vi "Untitled 1.vi"() -> ()   [LabVIEW 2016]
uses:
  Control 2.ctl
  Control 1.ctl
  <vilib>/Instr/_visa.llb/VISA Configure Serial Port (Instr).vi
panel:
  in  "Задать текущее положение нулевым":T1
  out "положение шд":T2 scale=-10.0..190.0
  out "минуты":string
  out "градусы, минуты":string
  in  "Установка минут":i32 min=0 max=11400
  out "положение в мин 1":i32
  in  "Stop двигатель":bool
  in  "Вернуться в нулевое положение":bool
  in  "Вращение по минутам -":bool
  in  "Вращение по минутам +":bool
  in  "stop":bool
  out "4":i32
  out "3":i32
  out "2":i32
  out "1":i32
  in  "Выберете порт":refnum<visa-resource-name>="COM1"
  # "Текущее\nположение:"
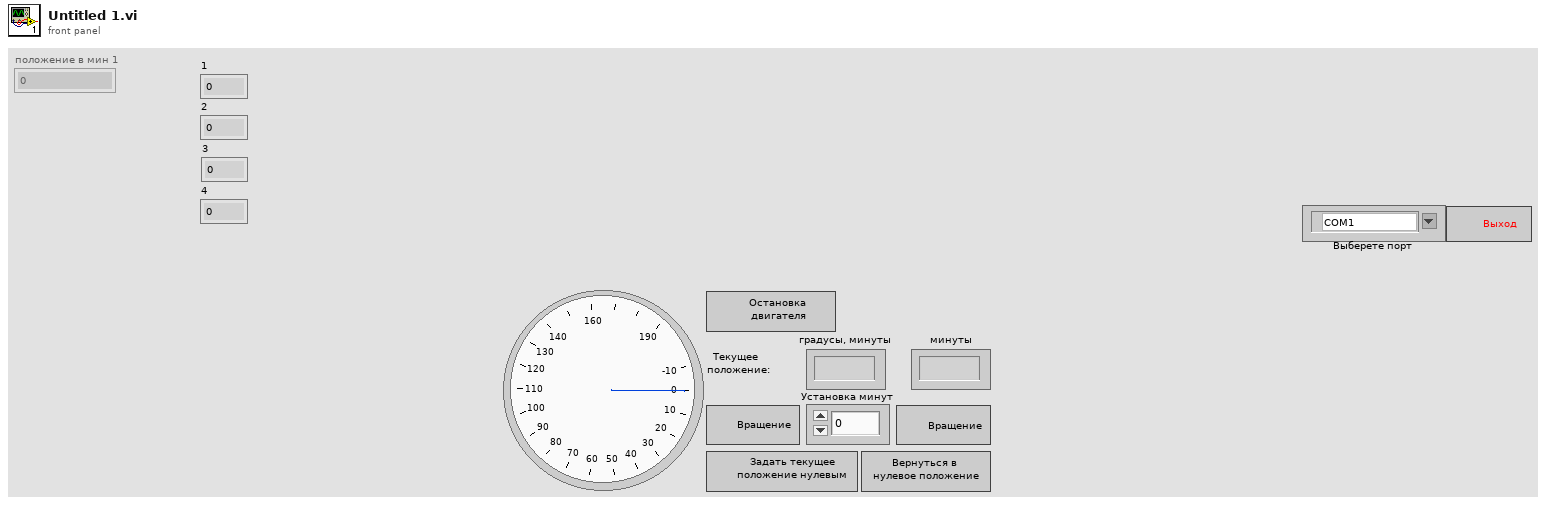
[diagram p1: front panel]
types:
  T1 = typedef "Control 1.ctl" = bool
  T2 = typedef "Control 2.ctl" = i32
  T3 = enum16{"open", "replace", "create", "open or create", "replace or create", "replace or create with confirmation"}
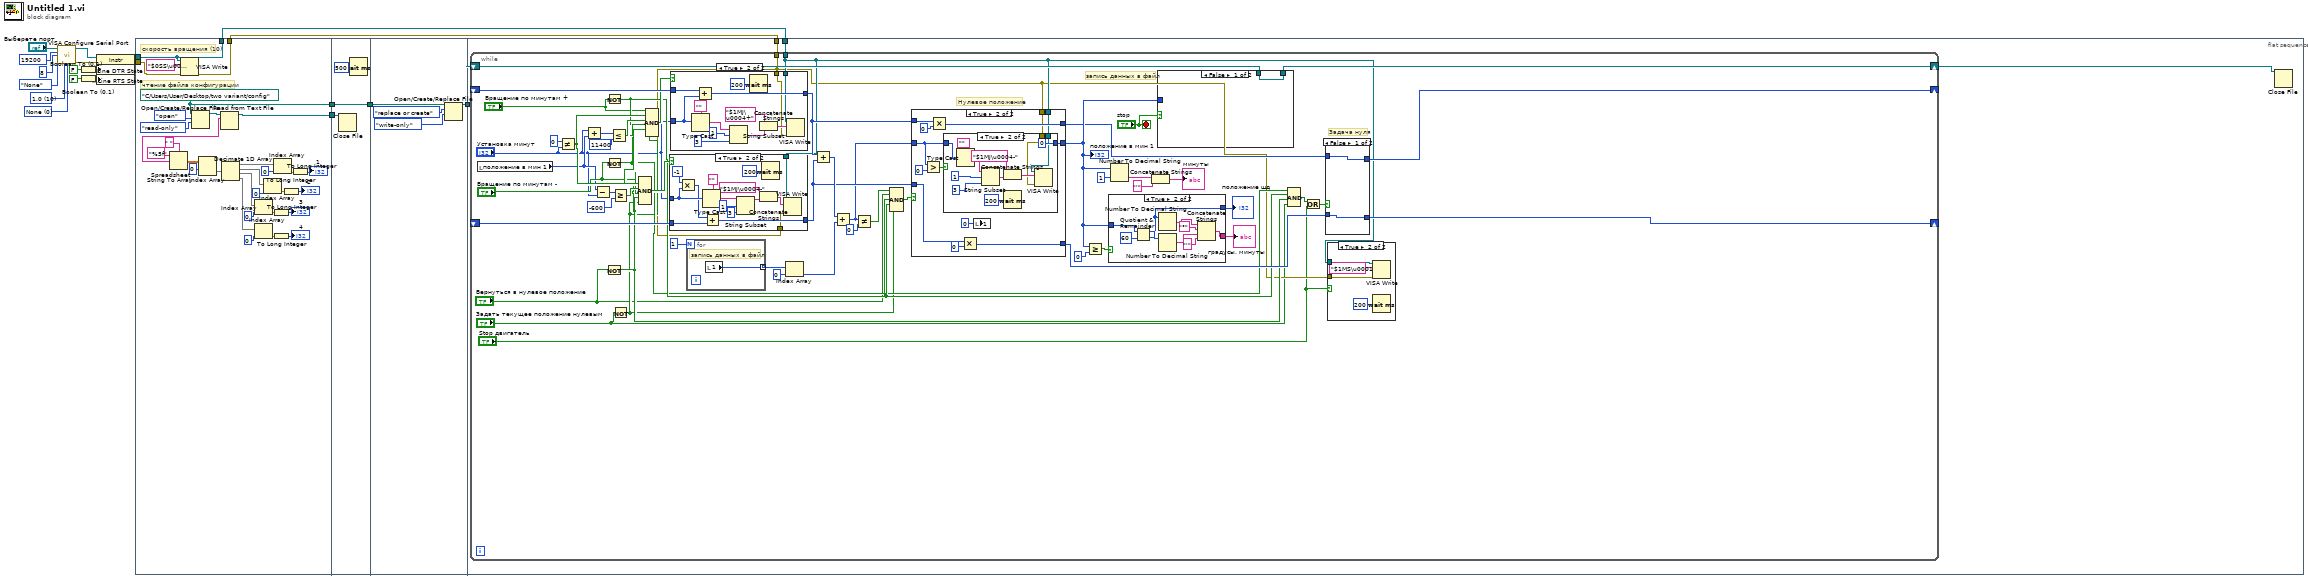
[diagram p0: block diagram]
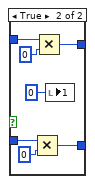
[diagram p3: hidden frame]
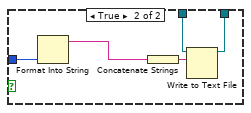
[diagram p4: hidden frame]
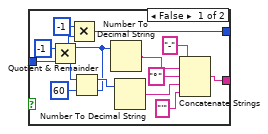
[diagram p5: hidden frame]
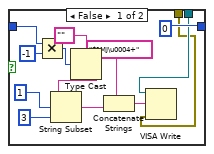
[diagram p7: hidden frame]
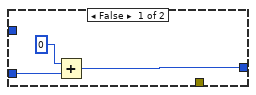
[diagram p8: hidden frame]
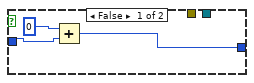
[diagram p9: hidden frame]
diagram:
  w9 = u16 0 items=["None"=0, "XON/XOFF"=1, "RTS/CTS"=2, "DTR/DSR"=4] ("Контроль переполнения")
  w10 = u16 10 items=["1.0"=10, "1.5"=15, "2.0"=20] ("Стоповый бит")
  w13 = u32 19200 items=["9600"=9600, "19200"=19200, "38400"=38400, "57600"=57600] ("Скорость обмена данными")
  n1 = call-poly "VISA Configure Serial Port"("VISA resource name"="Выберете порт", "baud rate (9600)"=w13, "data bits (8)"=u16 8 ("Число бит на символ"), "parity (0:none)"=enum16{"None", "Odd", "Even", "Mark", "Space"}."None" ("Контроль чётности"), "stop bits (10: 1 bit)"=w10, "flow control (0:none)"=w9) -> ("VISA resource name out"=w18:refnum<visa-resource-name>, "error out"=w17:errorcluster)  [unwired: 8 in]
  n2 = Boolean To (0,1)(Boolean=FALSE ("DTR Write")) -> (0, 1=w19:i16)
  n3 = Boolean To (0,1)(Boolean=FALSE ("DTR Write")) -> (0, 1=w20:i16)
  n4 = property class="Instr"(reference=w18, error in=w17, "Serial Settings:Modem Line Settings:Line DTR State"=w19, "Serial Settings:Modem Line Settings:Line RTS State"=w20) -> (reference out=w8:refnum<visa-resource-name>, error out=w7:errorcluster)
  n5 = flat-sequence {
    tunnel: w8 -> [w23]
    tunnel: w7 -> [w22]
    tunnel: [w24] -> w6
    tunnel: [w23] -> w1
    tunnel: [w22] -> w2
    tunnel: [w21] -> w5
    tunnel: w6 -> [w52]
    tunnel: w5 -> [w51]
    tunnel: [w51] -> w4
    tunnel: w4 -> [w55]
    tunnel: [w54] -> w3
    tunnel: w3 -> [w61]
    tunnel: w2 -> [w58]
    tunnel: w1 -> [w59]
    frame #0 {
      w21 = path "C:/Users/User/Desktop/two variant/config"
      # "чтение файла конфигурации"
      # "скорость вращения (10)"
      n6 = VISA Write(VISA resource name=w23, write buffer="$0SS\u0001\u0010", error in (no error)=w22) -> ()  [unwired: 3 out]
      n7 = Open/Create/Replace File(file path (use dialog)=w21, operation (0:open)=T3."open", access (0:read/write)=enum16{"read/write", "read-only", "write-only"}."read-only") -> (refnum out=w47:refnum<file>)  [unwired: 3 in, 2 out]
      n8 = Read from Text File(file (use dialog)=w47) -> (refnum out=w24:refnum<file>, text=w34:string)  [unwired: 3 in, 2 out]
      n9 = Spreadsheet String To Array(delimiter (Tab)=" ", format string="%5f", spreadsheet string=w34) -> (array=w44:dbl[][])  [unwired: 1 in]
      n10 = Index Array(array=w44, index (row)=0 ("index")) -> (element=w42:dbl[])  [unwired: 1 in]
      n11 = Decimate 1D Array(w42) -> (w39:dbl[], w30:dbl[], w29:dbl[], w25:dbl[])
      n12 = Index Array(array=w29, index=0) -> (element=w32:dbl)
      n13 = Index Array(array=w25, index=0) -> (element=w27:dbl)
      n14 = Index Array(array=w30, index=0) -> (element=w38:dbl)
      n15 = To Long Integer(number=w32) -> (32bit integer=→"3":i32)
      n16 = To Long Integer(number=w27) -> (32bit integer=→"4":i32)
      n17 = Index Array(array=w39, index=0) -> (element=w37:dbl)
      n18 = To Long Integer(number=w38) -> (32bit integer=→"2":i32)
      n19 = To Long Integer(number=w37) -> (32bit integer=→"1":i32)
    }
    frame #1 {
      n20 = Close File(refnum=w52) -> ()  [unwired: 1 in, 2 out]
      n21 = Wait (ms)(milliseconds to wait=u32 500) -> ()  [unwired: 1 out]
    }
    frame #2 {
      n22 = Open/Create/Replace File(file path (use dialog)=w55, operation (0:open)=T3."replace or create", access (0:read/write)=enum16{"read/write", "read-only", "write-only"}."write-only") -> (refnum out=w54:refnum<file>)  [unwired: 3 in, 2 out]
    }
    frame #3 {
      n23 = while {
        shift-right: [w85] -> w60
        shift-left: w61 -> [w86]
        shift-right: [w81] -> _
        shift-left: _ -> [w115]
        shift-right: [w80] -> _
        shift-left: _ -> [w109]
        tunnel: w59 -> [w73]
        tunnel: w58 -> [w72]
        stop <- "stop" stop-if-true
        # "Задача нуля"
        # "запись данных в файл"
        # "Нулевое положение"
        n24 = local read "положение в мин 1"() -> (w64:i32)
        n25 = Not Equal?(x=0 ("y"), y="Установка минут") -> (x != y?=w108:bool)
        n26 = Add(x="Установка минут", y=w64) -> (x+y=w113:i32)
        n27 = Subtract(x=w64, y="Установка минут") -> (x-y=w65:i32)
        n28 = Not(x="Вернуться в нулевое положение") -> (.not. x?=w79:bool)
        n29 = Not(x="Вращение по минутам +") -> (.not. x?=w78:bool)
        n30 = Not(x="Вращение по минутам -") -> (.not. x?=w77:bool)
        n31 = Less Or Equal?(x=w113, y=11400) -> (x <= y?=w112:bool)
        n32 = Greater Or Equal?(x=w65, y=-600) -> (x >= y?=w106:bool)
        n33 = Not(x="Задать текущее положение нулевым") -> (.not. x?=w76:T1)
        n34 = Compound Arithmetic op=AND("Вращение по минутам -", w108, w106, w78, w79, w76) -> (w105:T1)
        n35 = Compound Arithmetic op=AND("Вращение по минутам +", w108, w112, w77, w79, w76) -> (w110:T1)
        n36 = case shown="True" w105 {
          tunnel: [w201 w210] -> w95
          tunnel: "Установка минут" -> [_ w205]
          tunnel: w109 -> [w200 w206]
          tunnel: w73 -> [_ w208]
          tunnel: w72 -> [_ w207]
          frame False {
            n37 = Add(x=0, y=w200) -> (x+y=w201:i32)
          }
          frame True {
            n38 = Multiply(x=-1, y=w205) -> (x*y=w204:i32)
            n39 = Type Cast(type="", x=w205) -> (*(type *) &x=w213:string)
            n40 = Add(x=w204, y=w206) -> (x+y=w210:i32)
            n41 = String Subset(string=w213, offset (0)=1, length (rest)=3 ("length (rest)")) -> (substring=w212:string)
            n42 = Concatenate Strings("$1MJ\u0004-" ("write buffer"), w212) -> (w216:string)
            n43 = Wait (ms)(milliseconds to wait=u32 200) -> ()  [unwired: 1 out]
            n44 = VISA Write(VISA resource name=w208, write buffer=w216, error in (no error)=w207) -> ()  [unwired: 3 out]
          }
        }
        n45 = case shown="True" w110 {
          tunnel: [w219 w226] -> w96
          tunnel: "Установка минут" -> [_ w225]
          tunnel: w115 -> [w218 w222]
          tunnel: w73 -> [_ w224]
          tunnel: w72 -> [_ w223]
          frame False {
            n46 = Add(x=0, y=w218) -> (x+y=w219:i32)
          }
          frame True {
            n47 = Type Cast(type="", x=w225) -> (*(type *) &x=w229:string)
            n48 = Add(x=w222, y=w225) -> (x+y=w226:i32)
            n49 = String Subset(string=w229, offset (0)=1, length (rest)=3 ("length (rest)")) -> (substring=w228:string)
            n50 = Wait (ms)(milliseconds to wait=u32 200) -> ()  [unwired: 1 out]
            n51 = Concatenate Strings("$1MJ\u0004+" ("write buffer"), w228) -> (w232:string)
            n52 = VISA Write(VISA resource name=w224, write buffer=w232, error in (no error)=w223) -> ()  [unwired: 3 out]
          }
        }
        n53 = for {
          N: 1 -> [_]
          tunnel: [w199] -> w103 mode=indexing
          # "запись данных в файл"
          n54 = local read "1"() -> (w199:i32)
        }
        n55 = Index Array(array=w103, index=0) -> (element=w101:i32)
        n56 = Add(x=w96, y=w95) -> (x+y=w100:i32)
        n57 = Add(x=w100, y=w101) -> (x+y=w94:i32)
        n58 = Not Equal?(x=w94, y=0) -> (x != y?=w98:bool)
        n59 = Compound Arithmetic op=AND(w98, "Вернуться в нулевое положение", w77, w78, w76) -> (w97:T1)
        n60 = case shown="True" w97 {
          tunnel: [w158 w173] -> w84
          tunnel: [w160 w171] -> w83
          tunnel: [w159 w167] -> w82
          tunnel: w96 -> [w160 w165]
          tunnel: w95 -> [w159 w164]
          tunnel: w94 -> [w158 w163]
          tunnel: w73 -> [_ w162]
          tunnel: w72 -> [_ w161]
          frame False {
          }
          frame True {
            n61 = Greater?(x=w163, y=0) -> (0:w168:bool)
            n62 = Multiply(x=w165, y=0) -> (x*y=w171:i32)
            n63 = case shown="True" w168 {
              tunnel: [0 0] -> w173
              tunnel: w163 -> [w176 w190]
              tunnel: w162 -> [w175 w188]
              tunnel: w161 -> [w174 w189]
              frame False {
                n64 = Multiply(x=w176, y=-1) -> (x*y=w177:i32)
                n65 = Type Cast(type="", x=w177) -> (*(type *) &x=w182:string)
                n66 = String Subset(string=w182, offset (0)=1, length (rest)=3 ("length (rest)")) -> (substring=w181:string)
                n67 = Concatenate Strings("$1MJ\u0004+" ("write buffer"), w181) -> (w185:string)
                n68 = VISA Write(VISA resource name=w175, write buffer=w185, error in (no error)=w174) -> ()  [unwired: 3 out]
              }
              frame True {
                n69 = Type Cast(type="", x=w190) -> (*(type *) &x=w195:string)
                n70 = String Subset(string=w195, offset (0)=1, length (rest)=3 ("length (rest)")) -> (substring=w194:string)
                n71 = Concatenate Strings("$1MJ\u0004-" ("write buffer"), w194) -> (w191:string)
                n72 = Wait (ms)(milliseconds to wait=u32 200) -> ()  [unwired: 1 out]
                n73 = VISA Write(VISA resource name=w188, write buffer=w191, error in (no error)=w189) -> ()  [unwired: 3 out]
              }
            }
            n74 = Multiply(x=w164, y=0) -> (x*y=w167:i32)
            n75 = local write "1"(0 ("1")) -> ()
          }
        }
        "положение в мин 1" <- w84
        n76 = Greater Or Equal?(x=w84, y=0) -> (x >= y?=w93:bool)
        n77 = case shown="True" w93 {
          tunnel: [w145 w152] -> w87
          tunnel: [w136 w150] -> w67
          tunnel: w84 -> [w135 w149]
          frame False {
            n78 = Multiply(x=-1, y=w135) -> (x*y=w141:i32)
            n79 = Quotient & Remainder(x=w141, y=60) -> (x-y*floor(x/y)=w144:i32, floor(x/y)=w137:i32)
            n80 = Multiply(x=-1, y=w137) -> (x*y=w136:i32)
            n81 = Number To Decimal String(number=w137) -> (decimal integer string=w142:string)  [unwired: 1 in]
            n82 = Number To Decimal String(number=w144) -> (decimal integer string=w143:string)  [unwired: 1 in]
            n83 = Concatenate Strings("-" ("string"), w142, "°" ("string"), w143, "'" ("string")) -> (w145:string)
          }
          frame True {
            n84 = Quotient & Remainder(x=w149, y=60) -> (x-y*floor(x/y)=w151:i32, floor(x/y)=w150:i32)
            n85 = Number To Decimal String(number=w151) -> (decimal integer string=w153:string)  [unwired: 1 in]
            n86 = Number To Decimal String(number=w150) -> (decimal integer string=w154:string)  [unwired: 1 in]
            n87 = Concatenate Strings(w154, "°" ("string"), w153, "'" ("string")) -> (w152:string)
          }
        }
        "градусы, минуты" <- w87
        "положение шд" <- w67
        n88 = Number To Decimal String(number=w84, width (-)=i16 1) -> (decimal integer string=w90:string)
        n89 = Concatenate Strings(w90, "'" ("string")) -> (→"минуты":string)
        n90 = case shown="False" "stop" {
          tunnel: [w129 w134] -> w85
          tunnel: w86 -> [w129 w131]
          tunnel: w84 -> [_ w130]
          frame False {
          }
          frame True {
            n91 = Format Into String(w130) -> (resulting string=w132:string)  [unwired: 3 in, 1 out]
            n92 = Concatenate Strings(w132) -> (w133:string)
            n93 = Write to Text File(file (use dialog)=w131, text=w133) -> (refnum out=w134:refnum<file>)  [unwired: 2 in, 2 out]
          }
        }
        n94 = Compound Arithmetic op=AND(w77, w78, w79, "Задать текущее положение нулевым") -> (w74:T1)
        n95 = Or(x=w74, y="Stop двигатель") -> (x .or. y?=w75:T1)
        n96 = case shown="False" w75 {
          tunnel: [w121 w127] -> w81
          tunnel: w83 -> [w121 w128]
          tunnel: w82 -> [w120 w124]
          tunnel: [w120 w123] -> w80
          frame False {
          }
          frame True {
            n97 = Multiply(x=w124, y=0) -> (x*y=w123:i32)
            n98 = Multiply(x=w128, y=0) -> (x*y=w127:i32)
            n99 = local write "1"(0 ("1")) -> ()
          }
        }
        n100 = case shown="True" "Stop двигатель" {
          tunnel: w73 -> [_ w118]
          tunnel: w72 -> [_ w117]
          frame False {
          }
          frame True {
            n101 = Wait (ms)(milliseconds to wait=u32 200) -> ()  [unwired: 1 out]
            n102 = VISA Write(VISA resource name=w118, write buffer="$1MS\u0001", error in (no error)=w117) -> ()  [unwired: 3 out]
          }
        }
      }
      n103 = Close File(refnum=w60) -> ()  [unwired: 1 in, 2 out]
    }
  }
